vi "Roller Arm Position.vi"(10 "Right Pot":dbl, 11 "Left Pot":dbl) -> (1 "Right Closed?":bool, 2 "Left Closed?":bool, 3 "Portrait?":bool)   [LabVIEW 2014]
uses:
  Robot Global Data.vi
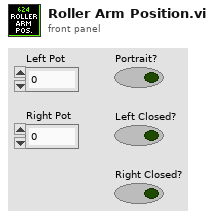
[diagram p1: front panel]
types:
  T1 = typedef "Dashboard Control Data.ctl" = cluster{"Cam Exposure":dbl, "Go to angle":dbl, "Steer PID Gains":cluster{"proportional gain (Kc)":dbl, "integral time (Ti, min)":dbl, "derivative time (Td, min)":dbl}, "Steer PID output Range":cluster{"output high":dbl, "output low":dbl}, "Pressure m \nValue":dbl, "Pressure b \nValue":dbl, "Strafe Timer\nWait":dbl, "Roller Command Cluster ":T2, "Elevator":T3, "Strafe Correct min X":dbl, "IMU Enable":bool, "Encoder Control":T5}
  T2 = typedef "Roller Control.ctl" = cluster{"Left Roller Speed":dbl, "Right Roller Speed":dbl, "Left Roller Speed Back":dbl, "Right Roller Speed Back":dbl, "Roller Align Decide Limit":u32, "Left Roller Speed Unload":dbl, "Right Roller Speed Unload":dbl, "Ping Dist Difference":dbl, "Ping In Dist":dbl, "Right Pot 0":dbl, "Pot Threshold":dbl, "Left Pot 0":dbl, "Manual 0s?":bool, "Right Pot Scale":dbl, "Left Pot Scale":dbl, "0 wait time":i32, "Reset?":bool}
  T3 = typedef "Elevator DB Control.ctl" = cluster{"PID Output Range":cluster{"output high":dbl, "output low":dbl}, "PID gains":cluster{"proportional gain (Kc)":dbl, "integral time (Ti, min)":dbl, "derivative time (Td, min)":dbl}, "Height Tolerance":dbl, " Encoder Constant":dbl, "Safe Mode Max Speed":dbl, "Eject Time":dbl, "Encoder Filter?":bool, "Zeroing Speed":dbl, "Presets":T4}
  T4 = typedef "Elevator Presets.ctl" = cluster{"Hold Tote":dbl, "Hold Trashcan":dbl, "Pickup 2 w/ Tote":dbl, "Pickup 2 w/ Trashcan":dbl, "Pickup 3 w/ Tote":dbl, "Pickup 3 w/ Trashcan":dbl, "Bottom":dbl, "Pickup 1 w/ Tote":dbl, "Pickup Trashcan":dbl, "Pickup 1 w/ Trashcan":dbl, "Eject":dbl}
  T5 = typedef "Encoder Control.ctl" = cluster{"Left Tick Constant":dbl, "Right Tick Constant":dbl, "Center Tick Constant":dbl, "Reset?":bool}
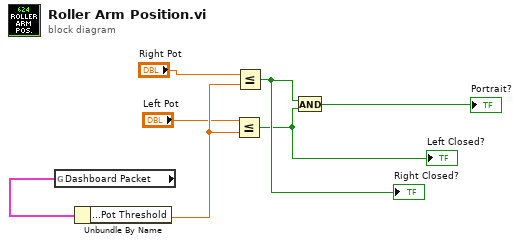
[diagram p0: block diagram]
diagram:
  n1 = global read "Robot Global Data.vi" "Dashboard Packet"() -> (w6:T1)
  n2 = Unbundle By Name(w6) -> ("Roller Command Cluster.Pot Threshold"=w7:dbl)
  n3 = Less Or Equal?(x="Left Pot", y=w7) -> (x <= y?=w2:bool)
  "Left Closed?" <- w2
  n4 = Less Or Equal?(x="Right Pot", y=w7) -> (x <= y?=w3:bool)
  "Right Closed?" <- w3
  n5 = And(x=w3, y=w2) -> (x .and. y?=→"Portrait?":bool)
